vi "WBPdetection.vi"() -> ()   [LabVIEW 2017, in "gVision.lvlib"]
uses:
  gVision.lvlib
panel:
  in  "yfov":dbl
  in  "xfov":dbl
  in  "tolerance":dbl
  in  "nominalHeight":dbl
  in  "nominalWidth":dbl
  in  "percent_size":dbl=0.4
  in  "File Path":path=path "C:/Users/hayde/OneDrive/Desktop/Research Code/201123_HDI_fiducial-20201128T195219Z-001/201123_HDI_fiducial/MH0111/fid_bl.png"
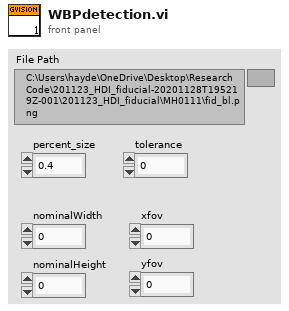
[diagram p1: front panel]
types:
  T1 = enum32{"Map Pixel Pointer", "Unmap Pixel Pointer", "Get Pixels Infos"}
  T2 = typedef "IMAQ Image.ctl" = refnum<image>
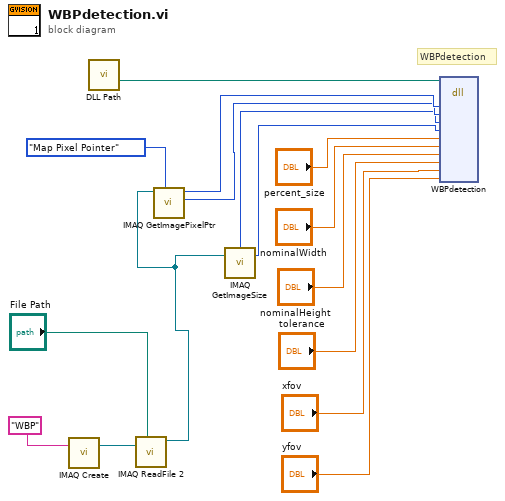
[diagram p0: block diagram]
diagram:
  # "WBPdetection"
  n1 = call "IMAQ Create"("Image Name"="WBP") -> ("New Image"=w14:T2)  [unwired: 4 in, 1 out]
  n2 = call "DLL Path.vi"() -> ("DLL Path"=w16:path)  [unwired: 5 in]
  n3 = call "IMAQ ReadFile 2"("File Path"="File Path", "Image"=w14) -> ("Image Out"=w11:T2)  [unwired: 5 in, 4 out]
  n4 = call "IMAQ GetImagePixelPtr"("Function"=T1."Map Pixel Pointer", "Image"=w11) -> ("LineWidth(Pixels)"=w9:i32, "Pixel Pointer out"=w10:u64)  [unwired: 4 in, 4 out]
  n5 = call "IMAQ GetImageSize"("Image"=w11) -> ("Y Resolution"=w7:i32, "X Resolution"=w8:i32)  [unwired: 3 in, 1 out]
  n6 = dll-call lib="?" fn="WBPdetection"(path in=w16, "img"=w10, "imgLineWidth"=w9, "imgWidth"=w8, "imgHeight"=w7, "percent_size"="percent_size", "nominalWidth"="nominalWidth", "nominalHeight"="nominalHeight", "tolerance"="tolerance", "xfov"="xfov", "yfov"="yfov") -> ()  [unwired: 13 in, 2 out]
